vi "New Footprint Segmented Log.vi"(6 "Size Check Period (1000 ms)":u32=1000, 8 "error in (no error)":errorcluster, 9 "Max Instances (-1: Unlimited)":i32=-1, 10 "Size Limit [bytes]":i64, 11 "Log File Specification":refnum<class "Log File Specification.lvclass">) -> (0 "error out":errorcluster, 3 "Footprint Segmented Log out":refnum<class "Footprint Segmented Log.lvclass">)   [LabVIEW 2012, in "Waveform Data Logger Engine.lvlib" / "Footprint Segmented Log.lvclass"]
doc: "Creates a new footprint-segmented log file, which specifies that a particular log file instance is closed after the log file reaches a certain size in bytes."
uses:
  Footprint Segmented Log.lvclass
  Shared/Classes/Log File Specifications/Log File Specification/Log File Specification.lvclass
  Segmented Log/Segmented Log Type.ctl
  Footprint Segmented Log.lvclass/Footprint Segmented Log.ctl
  Segmented Log/Segmented Log.lvclass/Segmented Log.ctl
  Segmented Log/Segmented Log.lvclass
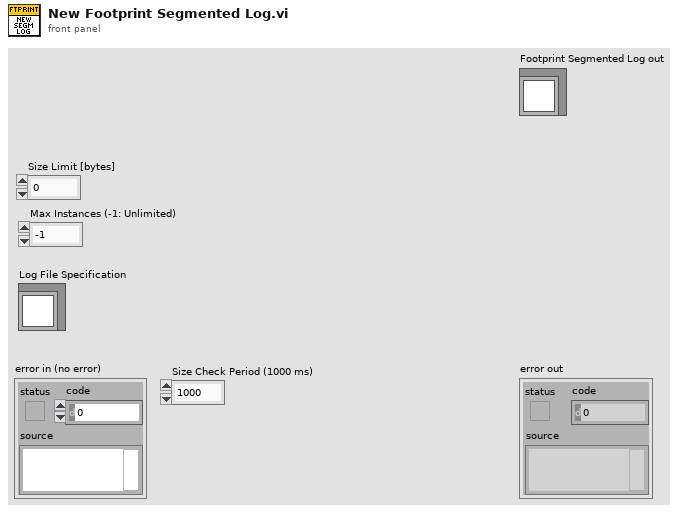
[diagram p1: front panel]
types:
  T1 = typedef "Waveform Data Logger Engine.lvlib/Segmented Log.lvclass/Segmented Log Type.ctl" = enum16{"No Limit", "Footprint", "Time"}
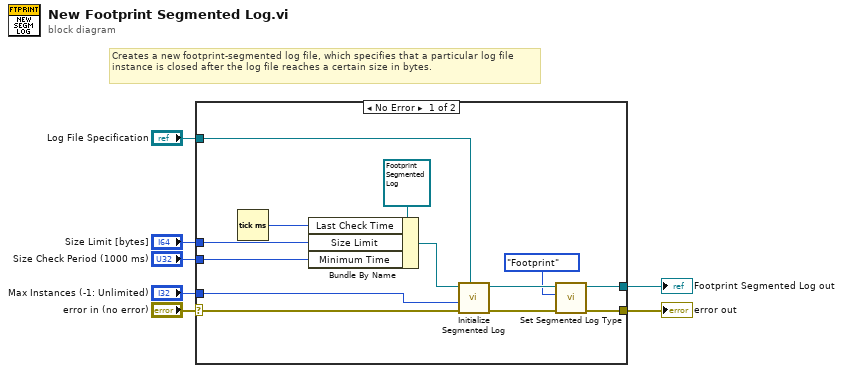
[diagram p0: block diagram]
diagram:
  # "Creates a new footprint-segmented log file, which specifies that a particular log file instance is closed after the log file reaches a certain size in bytes."
  n1 = case shown="No Error" "error in (no error)" {
    selector: "error in (no error)" -> [w20 w21]
    tunnel: [w8 w21] -> w6
    tunnel: [w9 _] -> w5
    tunnel: "Size Limit [bytes]" -> [w18 _]
    tunnel: "Log File Specification" -> [w17 _]
    tunnel: "Max Instances (-1: Unlimited)" -> [w16 _]
    tunnel: "Size Check Period (1000 ms)" -> [w14 _]
    frame No Error {
      n2 = Tick Count (ms)() -> (millisecond timer value=w15:u32)
      n3 = Bundle By Name(cluster=refnum<class "Footprint Segmented Log.lvclass"> refnum ("Footprint Segmented Log in"), "Last Check Time"=w15, "Size Limit"=w18, "Minimum Time"=w14) -> (w19:refnum<class "Footprint Segmented Log.lvclass">)
      n4 = call "Initialize Segmented Log.vi"("Log File Specification"=w17, "error in (no error)"=w20, "Max Instances (1)"=w16, "Segmented Log in"=w19) -> ("error out"=w11:errorcluster, "Segmented Log out"=w12:refnum<class "Footprint Segmented Log.lvclass">)  [unwired: 6 in]
      n5 = call "Set Segmented Log Type.vi"("error in (no error)"=w11, "Segmented Log Type"=Segmented_Log_Type."Footprint", "Segmented Log in"=w12) -> ("error out"=w8:errorcluster, "Segmented Log out"=w9:refnum<class "Footprint Segmented Log.lvclass">)  [unwired: 7 in]
    }
    frame Error {
    }
  }
  "error out" <- w6
  "Footprint Segmented Log out" <- w5
